vi "Robot Arm Cheval.vi"(7 "Motor Speed":dbl, 8 "Abort":bool, 9 "Limit Switch Shoulder":bool, 10 "Limit Switch Elbow":bool, 11 "Start Cheval":bool) -> (0 "Done":bool=TRUE, 1 "Arcada Drive":T1, 2 "Set Shoulder":dbl, 3 "Set Elbow":dbl)   [LabVIEW 2015]
uses:
  cheval_auto_states.ctl
  Sensors.vi
panel:
  out "Limit Switch Elbow 2":bool
  out "Limit Switch Shoulder 2":bool
  in  "Kd":dbl=0.005
  in  "Kp":dbl=0.05
  in  "Ki":dbl
  in  "Drive Time":dbl
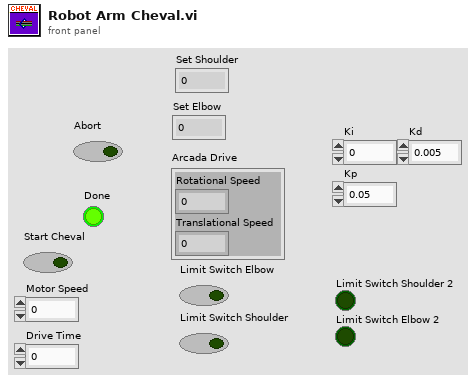
[diagram p1: front panel]
types:
  T1 = cluster{"Rotational Speed":dbl, "Translational Speed":dbl}
  T2 = typedef "cheval_auto_states.ctl" = enum16{"Ready", "Arm Down", "Arm To Bottom", "Drive Over", "Arm to rest", "stop"}
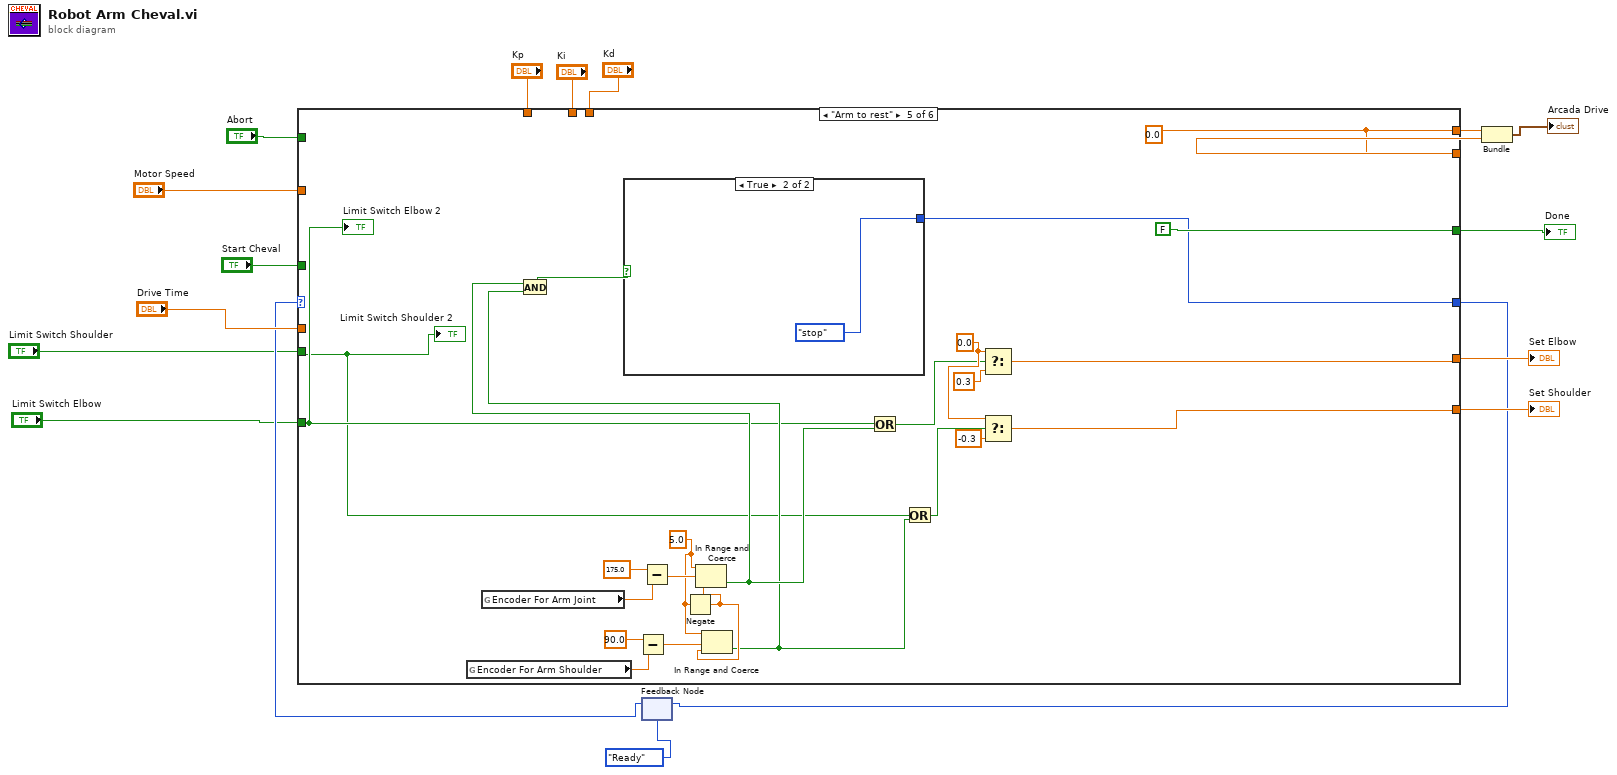
[diagram p0: block diagram]
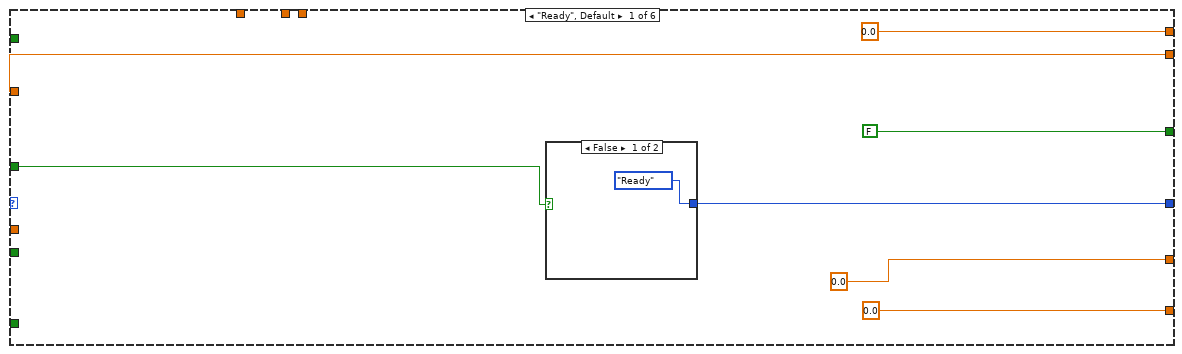
[diagram p2: hidden frame]
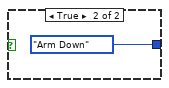
[diagram p3: hidden frame]
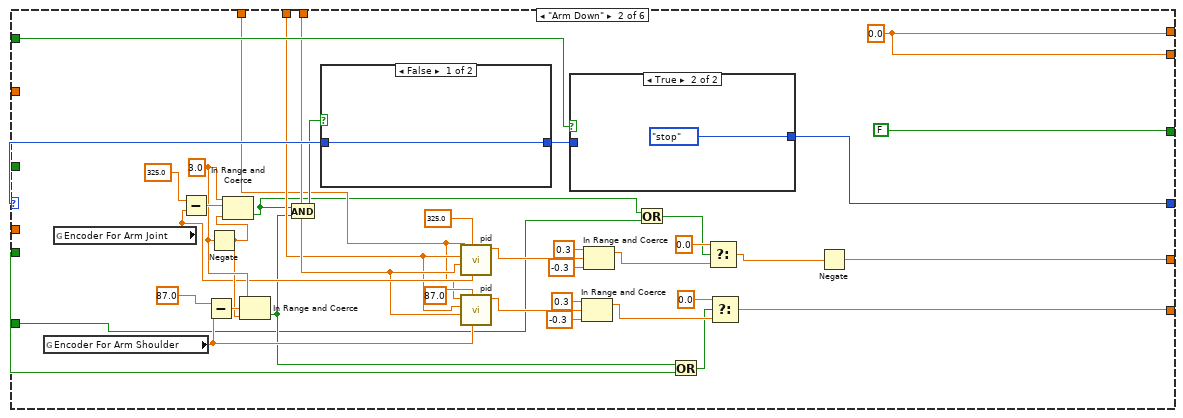
[diagram p4: hidden frame]
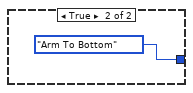
[diagram p5: hidden frame]
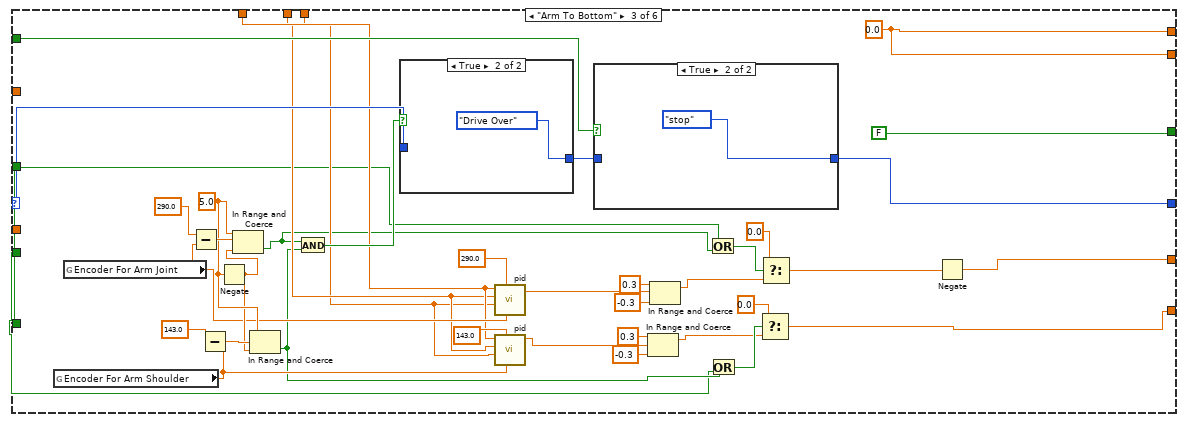
[diagram p7: hidden frame]
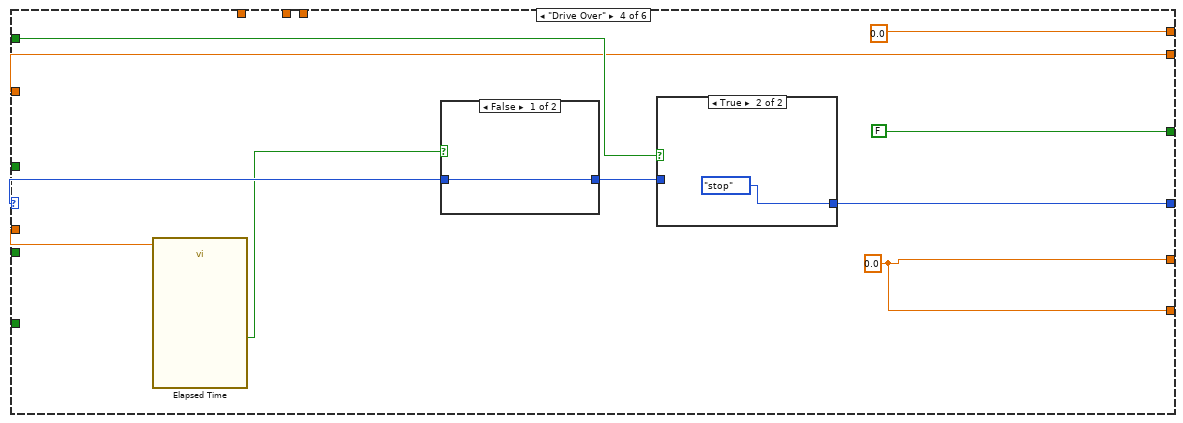
[diagram p10: hidden frame]
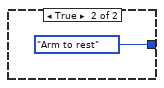
[diagram p12: hidden frame]
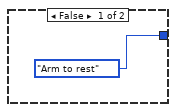
[diagram p13: hidden frame]
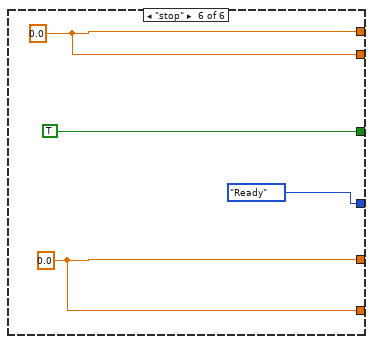
[diagram p14: hidden frame]
diagram:
  n1 = feedback #1(cheval_auto_states."Ready") -> (w9:T2)
  n2 = case shown="\"Arm to rest\"" w9 {
    selector: w9 -> [_ w63 w109 w120 _ _]
    tunnel: [w25 w64 w107 w121 w148 cheval_auto_states."Ready"] -> w8
    tunnel: "Abort" -> [_ w66 w106 w123 _ _]
    tunnel: "Motor Speed" -> [w24 _ _ w119 _ _]
    tunnel: "Drive Time" -> [_ _ _ w116 _ _]
    tunnel: [0.0 w50 w93 0.0 w128 w155] -> w15
    tunnel: [FALSE FALSE FALSE FALSE FALSE TRUE] -> w13
    tunnel: [0.0 ("Set Motor at S") w28 w71 w114 w144 w154] -> w12
    tunnel: [0.0 ("Set Motor at 1") w30 w72 w114 w143 w154] -> w11
    tunnel: [w24 w50 w93 w119 w128 w155] -> w7
    tunnel: "Limit Switch Shoulder" -> [_ w35 w80 _ w129 _]
    tunnel: "Limit Switch Elbow" -> [_ w32 w81 _ w130 _]
    tunnel: "Kp" -> [_ w41 w86 _ _ _]
    tunnel: "Ki" -> [_ w42 w85 _ _ _]
    tunnel: "Kd" -> [_ w43 w84 _ _ _]
    tunnel: "Start Cheval" -> [w19 _ _ _ _ _]
    frame "Ready", Default {
      n3 = case shown="False" w19 {
        tunnel: [cheval_auto_states."Ready" cheval_auto_states."Arm Down"] -> w25
        frame False {
        }
        frame True {
        }
      }
    }
    frame "Arm Down" {
      w54 = 3.0
      w50 = 0.0
      n4 = global read "Sensors.vi" "Encoder For Arm Shoulder"() -> (w52:dbl)
      n5 = global read "Sensors.vi" "Encoder For Arm Joint"() -> (w51:dbl)
      n6 = Subtract(x=325.0 ("setpoint"), y=w51) -> (x-y=w56:dbl)
      n7 = Subtract(x=87.0 ("setpoint"), y=w52) -> (x-y=w59:dbl)
      n8 = Negate(x=w54) -> (-x=w53:dbl)
      n9 = In Range and Coerce(upper limit=w54, x=w56, lower limit=w53) -> (In Range?=w31:bool)  [unwired: 1 out]
      n10 = In Range and Coerce(upper limit=w54, x=w59, lower limit=w53) -> (In Range?=w36:bool)  [unwired: 1 out]
      n11 = And(x=w31, y=w36) -> (x .and. y?=w57:bool)
      n12 = case shown="False" w57 {
        tunnel: [w67 cheval_auto_states."Arm To Bottom"] -> w65
        tunnel: w63 -> [w67 _]
        frame False {
        }
        frame True {
        }
      }
      n13 = call "pid.vi"("y"=w51, "setpoint"=325.0, "kd"=w43, "ki"=w42, "kp"=w41) -> ("Motor Command"=w49:dbl)  [unwired: 6 in]
      n14 = call "pid.vi"("y"=w52, "setpoint"=87.0, "kd"=w43, "ki"=w42, "kp"=w41) -> ("Motor Command"=w44:dbl)  [unwired: 6 in]
      n15 = case shown="True" w66 {
        tunnel: w65 -> [w69 _]
        tunnel: [w69 cheval_auto_states."stop"] -> w64
        frame False {
        }
        frame True {
        }
      }
      n16 = In Range and Coerce(upper limit=0.3, x=w44, lower limit=-0.3) -> (coerced(x)=w38:dbl)  [unwired: 1 out]
      n17 = In Range and Coerce(upper limit=0.3, x=w49, lower limit=-0.3) -> (coerced(x)=w40:dbl)  [unwired: 1 out]
      n18 = Or(x=w31, y=w32) -> (x .or. y?=w33:bool)
      n19 = Or(x=w36, y=w35) -> (x .or. y?=w34:bool)
      n20 = Select(t=0.0, s=w33, f=w40) -> (s? t:f=w29:dbl)
      n21 = Select(t=0.0, s=w34, f=w38) -> (s? t:f=w30:dbl)
      n22 = Negate(x=w29) -> (-x=w28:dbl)
    }
    frame "Arm To Bottom" {
      w100 = 5.0
      w93 = 0.0
      n23 = global read "Sensors.vi" "Encoder For Arm Shoulder"() -> (w94:dbl)
      n24 = global read "Sensors.vi" "Encoder For Arm Joint"() -> (w95:dbl)
      n25 = Subtract(x=290.0 ("setpoint"), y=w95) -> (x-y=w102:dbl)
      n26 = Subtract(x=143.0 ("setpoint"), y=w94) -> (x-y=w104:dbl)
      n27 = Negate(x=w100) -> (-x=w99:dbl)
      n28 = In Range and Coerce(upper limit=w100, x=w102, lower limit=w99) -> (In Range?=w82:bool)  [unwired: 1 out]
      n29 = In Range and Coerce(upper limit=w100, x=w104, lower limit=w99) -> (In Range?=w83:bool)  [unwired: 1 out]
      n30 = And(x=w82, y=w83) -> (x .and. y?=w98:bool)
      n31 = case shown="True" w98 {
        tunnel: w109 -> [w112 _]
        tunnel: [w112 cheval_auto_states."Drive Over"] -> w108
        frame False {
        }
        frame True {
        }
      }
      n32 = call "pid.vi"("y"=w95, "setpoint"=290.0, "kd"=w84, "ki"=w85, "kp"=w86) -> ("Motor Command"=w88:dbl)  [unwired: 6 in]
      n33 = call "pid.vi"("y"=w94, "setpoint"=143.0, "kd"=w84, "ki"=w85, "kp"=w86) -> ("Motor Command"=w87:dbl)  [unwired: 6 in]
      n34 = case shown="True" w106 {
        tunnel: w108 -> [w110 _]
        tunnel: [w110 cheval_auto_states."stop"] -> w107
        frame False {
        }
        frame True {
        }
      }
      n35 = In Range and Coerce(upper limit=0.3, x=w87, lower limit=-0.3) -> (coerced(x)=w75:dbl)  [unwired: 1 out]
      n36 = In Range and Coerce(upper limit=0.3, x=w88, lower limit=-0.3) -> (coerced(x)=w74:dbl)  [unwired: 1 out]
      n37 = Or(x=w81, y=w82) -> (x .or. y?=w79:bool)
      n38 = Or(x=w83, y=w80) -> (x .or. y?=w78:bool)
      n39 = Select(t=0.0, s=w78, f=w75) -> (s? t:f=w72:dbl)
      n40 = Select(t=0.0, s=w79, f=w74) -> (s? t:f=w73:dbl)
      n41 = Negate(x=w73) -> (-x=w71:dbl)
    }
    frame "Drive Over" {
      w114 = 0.0
      n42 = call "Elapsed Time"("Time Target (s)"=w116) -> ("Time has Elapsed"=w115:bool)  [unwired: 11 in, 7 out]
      n43 = case shown="False" w115 {
        tunnel: [w126 cheval_auto_states."Arm to rest"] -> w122
        tunnel: w120 -> [w126 _]
        frame False {
        }
        frame True {
        }
      }
      n44 = case shown="True" w123 {
        tunnel: w122 -> [w124 _]
        tunnel: [w124 cheval_auto_states."stop"] -> w121
        frame False {
        }
        frame True {
        }
      }
    }
    frame "Arm to rest" {
      w136 = 5.0
      w145 = 0.0
      w128 = 0.0
      n45 = global read "Sensors.vi" "Encoder For Arm Shoulder"() -> (w140:dbl)
      n46 = global read "Sensors.vi" "Encoder For Arm Joint"() -> (w141:dbl)
      n47 = Subtract(x=90.0, y=w140) -> (x-y=w137:dbl)
      n48 = Subtract(x=175.0, y=w141) -> (x-y=w138:dbl)
      n49 = Negate(x=w136) -> (-x=w135:dbl)
      n50 = In Range and Coerce(upper limit=w136, x=w138, lower limit=w135) -> (In Range?=w132:bool)  [unwired: 1 out]
      n51 = In Range and Coerce(upper limit=w136, x=w137, lower limit=w135) -> (In Range?=w131:bool)  [unwired: 1 out]
      n52 = And(x=w132, y=w131) -> (x .and. y?=w149:bool)
      n53 = case shown="True" w149 {
        tunnel: [cheval_auto_states."Arm to rest" cheval_auto_states."stop"] -> w148
        frame False {
        }
        frame True {
        }
      }
      n54 = Or(x=w130, y=w132) -> (x .or. y?=w133:bool)
      n55 = Or(x=w129, y=w131) -> (x .or. y?=w134:bool)
      n56 = Select(t=w145, s=w133, f=0.3) -> (s? t:f=w144:dbl)
      n57 = Select(t=w145, s=w134, f=-0.3) -> (s? t:f=w143:dbl)
      "Limit Switch Shoulder 2" <- w129
      "Limit Switch Elbow 2" <- w130
    }
    frame "stop" {
      w154 = 0.0
      w155 = 0.0
    }
  }
  "Done" <- w13
  "Set Elbow" <- w12
  "Set Shoulder" <- w11
  n58 = feedback-in #1(w8) -> ()
  n59 = Bundle(w15, "Motor Speed"=w7) -> (→"Arcada Drive":cluster{dbl, "Motor Speed":dbl})  [unwired: 1 in]
